vi "Untitled 2.vi"() -> ()   [LabVIEW 2016]
doc: "Приложение для управления четырьмя шаговыми двигателями. Обратной связи с двигателями не имеется."
uses:
  Control 2.ctl
  Control 1.ctl
  Control 3.ctl
  Control 4.ctl
  Control 5.ctl
  <vilib>/Instr/_visa.llb/VISA Configure Serial Port (Instr).vi
panel:
  in  "Stop двигатель 4":T1
  in  "Блокировать счётчик №4":T2
  out "text4":string
  in  "Задать текущее положение нулевым 4":T3
  out "положение шд 4":T4 scale=-10.0..190.0
  in  "Установка шага вращения":i32=1 min=0 max=11400
  in  "Вернуться в нулевое положение 4":bool
  in  "Вращение по минутам - 4":bool
  in  "Вращение по минутам + 4":bool
  out "минуты":string
  out "градусы, минуты":string
  out "положение в мин 4":i32
  in  "stop":T5
  in  "Stop двигатель 3":T1
  in  "Блокировать трубку №3":T2
  out "text3":string
  in  "Задать текущее положение нулевым 3":T3
  out "положение шд 3":T4 scale=-10.0..190.0
  in  "Установка шага вращения":i32=1 min=0 max=11400
  in  "Вернуться в нулевое положение 3":bool
  in  "Вращение по минутам - 3":bool
  in  "Вращение по минутам + 3":bool
  out "минуты":string
  out "градусы, минуты":string
  out "положение в мин 3":i32
  in  "Блокировать стол №2":T2
  out "text2":string
  in  "Stop двигатель 2":T1
  out "положение в мин 2":i32
  out "градусы, минуты":string
  out "минуты":string
  in  "Вращение по минутам + 2":bool
  in  "Вращение по минутам - 2":bool
  in  "Вернуться в нулевое положение 2":bool
  in  "Установка шага вращения":i32=1 min=0 max=11400
  out "положение шд 2":T4 scale=-10.0..190.0
  in  "Задать текущее положение нулевым 2":T3
  in  "Блокировать зеркало №1":bool
  in  "Задать текущее положение нулевым":T3
  out "положение шд":T4 scale=-10.0..190.0
  out "минуты":string
  out "градусы, минуты":string
  in  "Установка шага вращения":i32=1 min=0 max=11400
  out "положение в мин 1":i32
  in  "Stop двигатель":bool
  in  "Вернуться в нулевое положение":bool
  in  "Вращение по минутам -":bool
  in  "Вращение по минутам +":bool
  out "4":i32
  out "3":i32
  out "2":i32
  out "1":i32
  in  "Выберете порт":refnum<visa-resource-name>="COM1"
  # "Поворотный стол №2"
  # "Зеркало №1"
  # "Текущее\nположение"
  # "Текущее\nположение"
  # "Счётчик №4"
  # "Рентгеновская трубка №3"
  # "Текущее\nположение"
  # "Текущее\nположение"
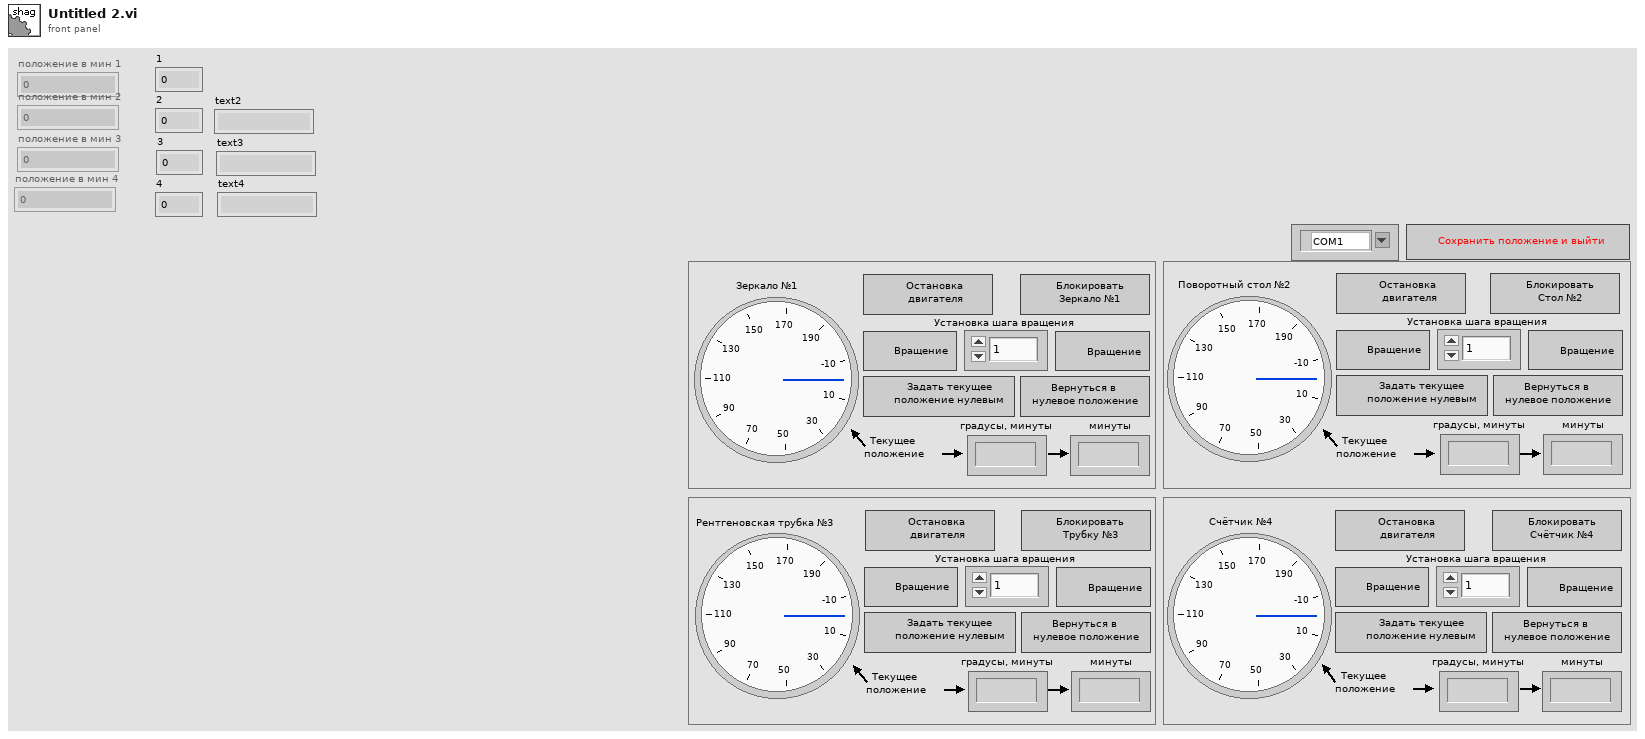
[diagram p1: front panel]
types:
  T1 = typedef "Control 3.ctl" = bool
  T2 = typedef "Control 4.ctl" = bool
  T3 = typedef "Control 1.ctl" = bool
  T4 = typedef "Control 2.ctl" = i32
  T5 = typedef "Control 5.ctl" = bool
  T6 = enum16{"open", "replace", "create", "open or create", "replace or create", "replace or create with confirmation"}
  T7 = enum8{"Enabled", "Disabled", "Disabled and Grayed Out"}
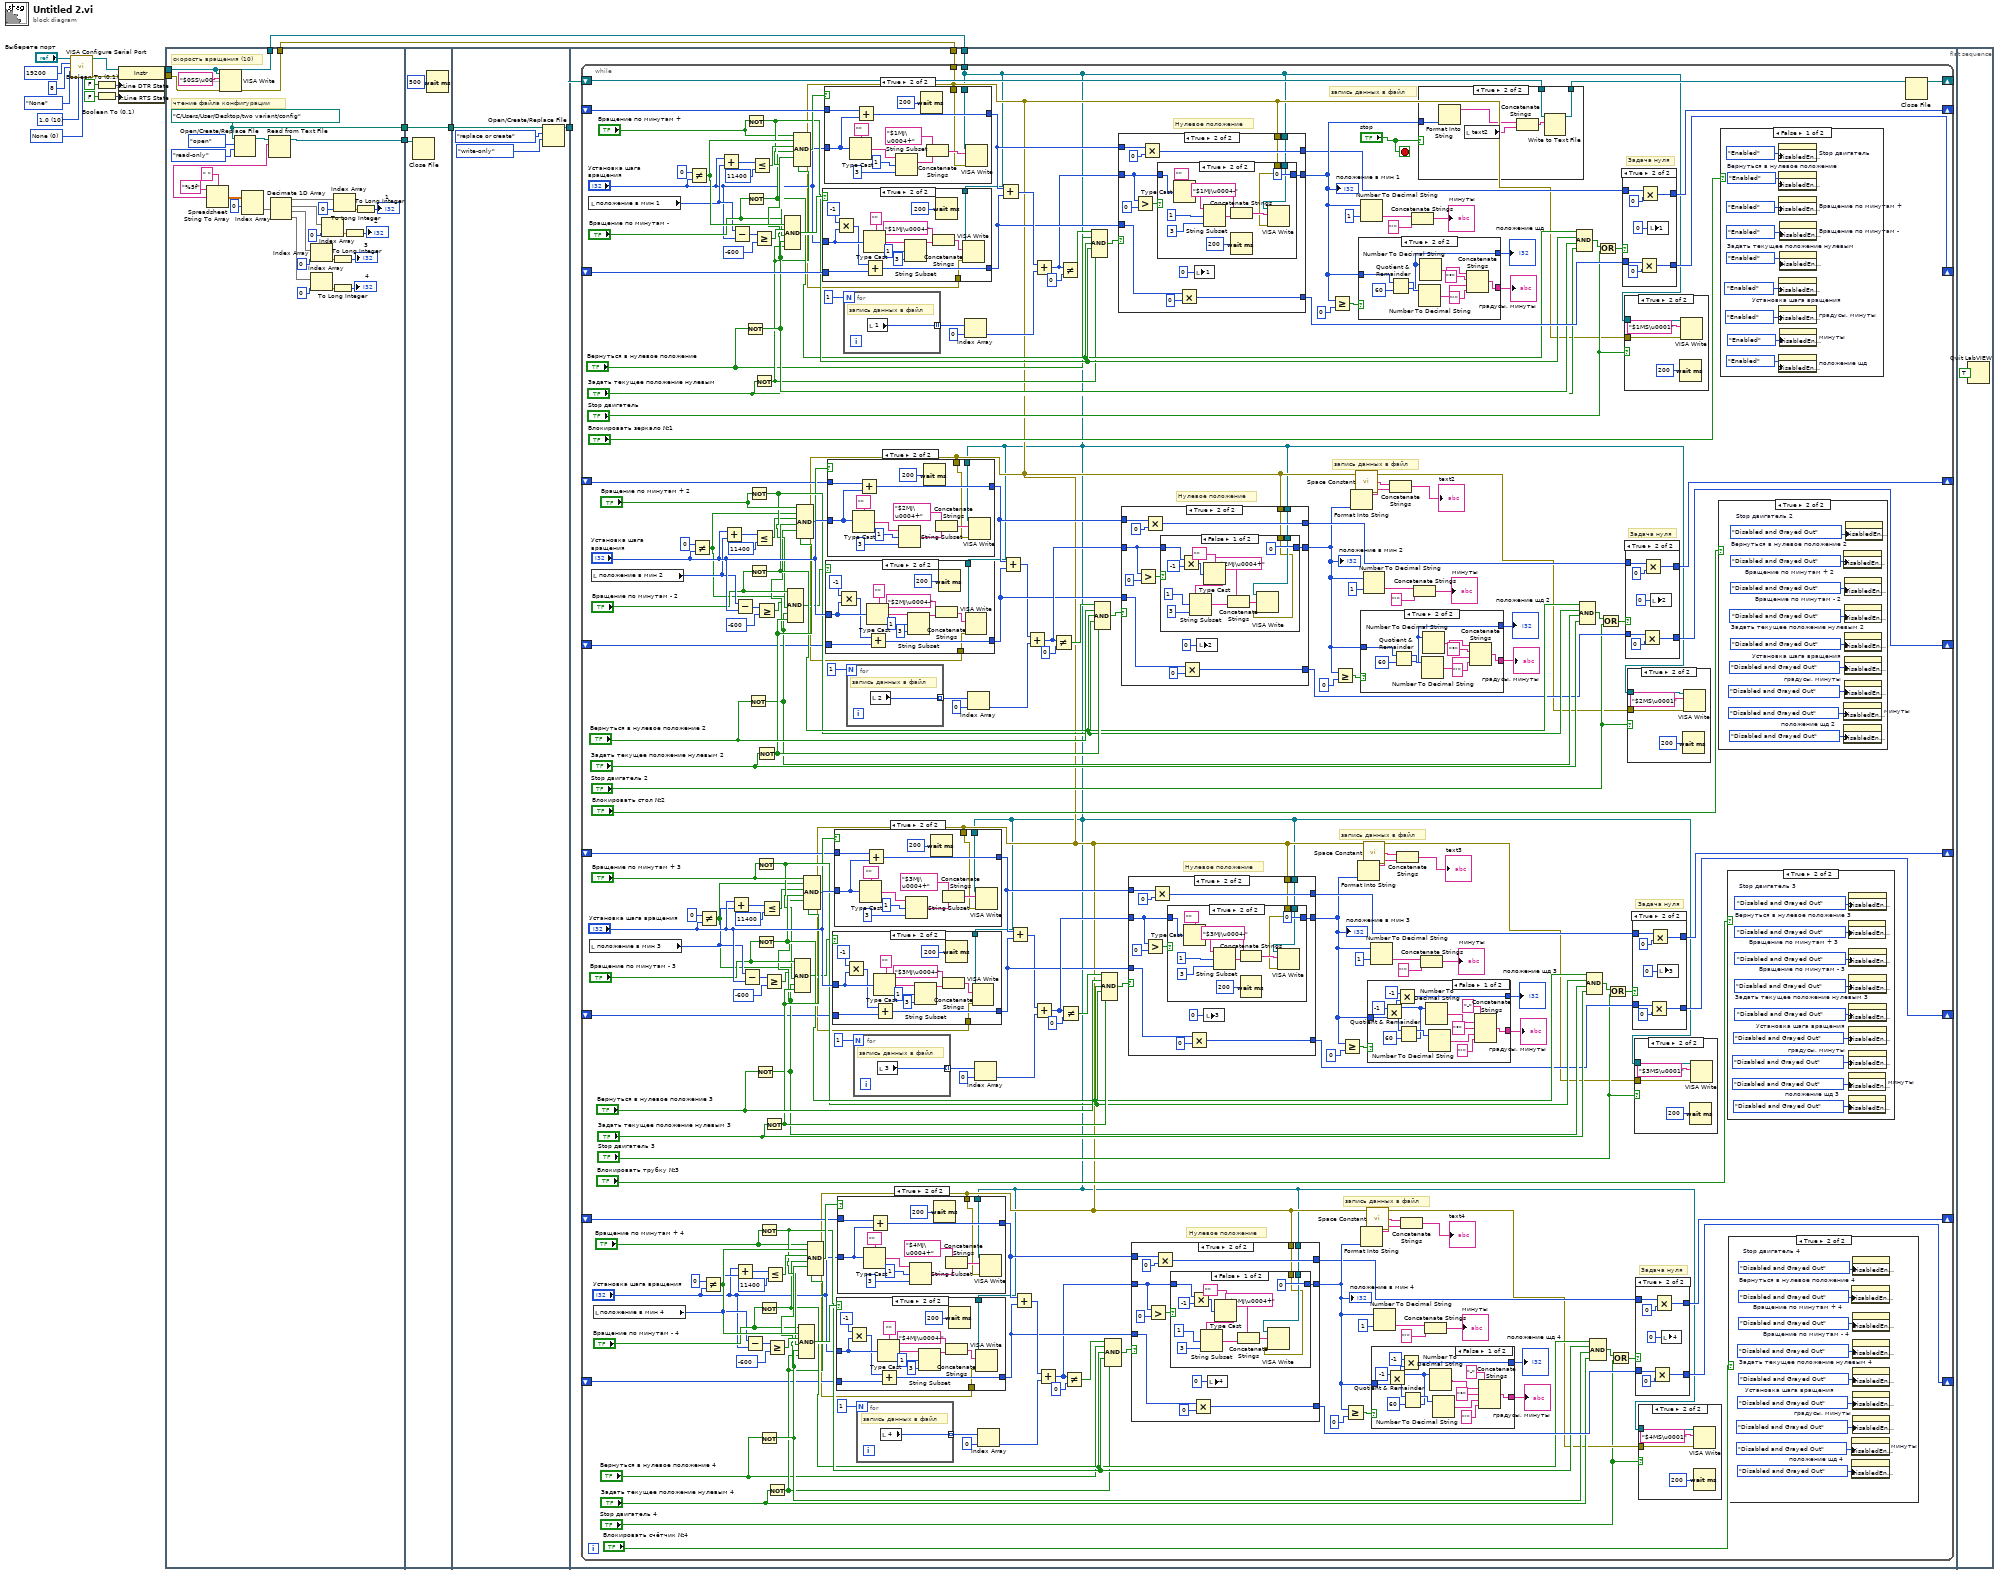
[diagram p0: block diagram]
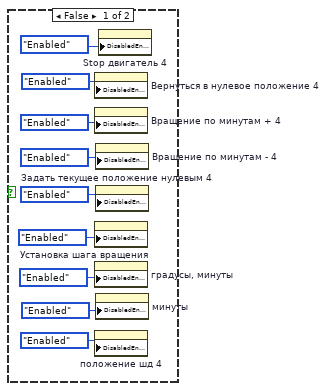
[diagram p2: hidden frame]
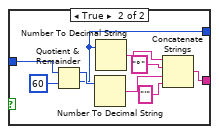
[diagram p5: hidden frame]
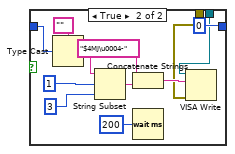
[diagram p7: hidden frame]
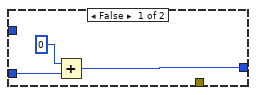
[diagram p8: hidden frame]
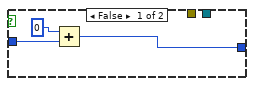
[diagram p9: hidden frame]
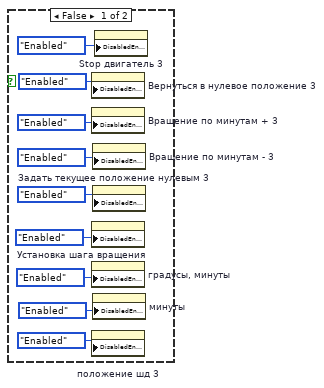
[diagram p10: hidden frame]
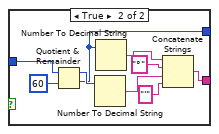
[diagram p13: hidden frame]
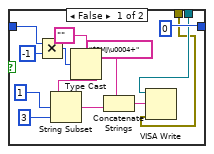
[diagram p15: hidden frame]
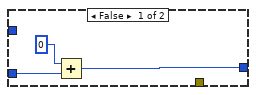
[diagram p16: hidden frame]
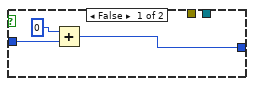
[diagram p17: hidden frame]
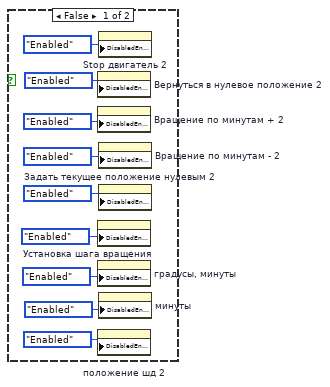
[diagram p18: hidden frame]
diagram:
  w9 = u16 0 items=["None"=0, "XON/XOFF"=1, "RTS/CTS"=2, "DTR/DSR"=4] ("Контроль переполнения")
  w10 = u16 10 items=["1.0"=10, "1.5"=15, "2.0"=20] ("Стоповый бит")
  w13 = u32 19200 items=["9600"=9600, "19200"=19200, "38400"=38400, "57600"=57600] ("Скорость обмена данными")
  n1 = call-poly "VISA Configure Serial Port"("VISA resource name"="Выберете порт", "baud rate (9600)"=w13, "data bits (8)"=u16 8 ("Число бит на символ"), "parity (0:none)"=enum16{"None", "Odd", "Even", "Mark", "Space"}."None" ("Контроль чётности"), "stop bits (10: 1 bit)"=w10, "flow control (0:none)"=w9) -> ("VISA resource name out"=w18:refnum<visa-resource-name>, "error out"=w17:errorcluster)  [unwired: 8 in]
  n2 = Boolean To (0,1)(Boolean=FALSE ("DTR Write")) -> (0, 1=w19:i16)
  n3 = Boolean To (0,1)(Boolean=FALSE ("DTR Write")) -> (0, 1=w20:i16)
  n4 = property class="Instr"(reference=w18, error in=w17, "Serial Settings:Modem Line Settings:Line DTR State"=w19, "Serial Settings:Modem Line Settings:Line RTS State"=w20) -> (reference out=w8:refnum<visa-resource-name>, error out=w7:errorcluster)
  n5 = flat-sequence {
    tunnel: w8 -> [w23]
    tunnel: w7 -> [w22]
    tunnel: [w24] -> w6
    tunnel: [w23] -> w1
    tunnel: [w22] -> w2
    tunnel: [w21] -> w5
    tunnel: w6 -> [w52]
    tunnel: w5 -> [w51]
    tunnel: [w51] -> w4
    tunnel: w4 -> [w55]
    tunnel: [w54] -> w3
    tunnel: w3 -> [w61]
    tunnel: w2 -> [w58]
    tunnel: w1 -> [w59]
    frame #0 {
      w21 = path "C:/Users/User/Desktop/two variant/config"
      # "чтение файла конфигурации"
      # "скорость вращения (10)"
      n6 = VISA Write(VISA resource name=w23, write buffer="$0SS\u0001\u0010", error in (no error)=w22) -> ()  [unwired: 3 out]
      n7 = Open/Create/Replace File(file path (use dialog)=w21, operation (0:open)=T6."open", access (0:read/write)=enum16{"read/write", "read-only", "write-only"}."read-only") -> (refnum out=w47:refnum<file>)  [unwired: 3 in, 2 out]
      n8 = Read from Text File(file (use dialog)=w47) -> (refnum out=w24:refnum<file>, text=w34:string)  [unwired: 3 in, 2 out]
      n9 = Spreadsheet String To Array(delimiter (Tab)=" ", format string="%5f", spreadsheet string=w34) -> (array=w44:dbl[][])  [unwired: 1 in]
      n10 = Index Array(array=w44, index (row)=0 ("index")) -> (element=w42:dbl[])  [unwired: 1 in]
      n11 = Decimate 1D Array(w42) -> (w39:dbl[], w30:dbl[], w29:dbl[], w25:dbl[])
      n12 = Index Array(array=w29, index=0) -> (element=w32:dbl)
      n13 = Index Array(array=w25, index=0) -> (element=w27:dbl)
      n14 = Index Array(array=w30, index=0) -> (element=w38:dbl)
      n15 = To Long Integer(number=w32) -> (32bit integer=→"3":i32)
      n16 = To Long Integer(number=w27) -> (32bit integer=→"4":i32)
      n17 = Index Array(array=w39, index=0) -> (element=w37:dbl)
      n18 = To Long Integer(number=w38) -> (32bit integer=→"2":i32)
      n19 = To Long Integer(number=w37) -> (32bit integer=→"1":i32)
    }
    frame #1 {
      n20 = Close File(refnum=w52) -> ()  [unwired: 1 in, 2 out]
      n21 = Wait (ms)(milliseconds to wait=u32 500) -> ()  [unwired: 1 out]
    }
    frame #2 {
      n22 = Open/Create/Replace File(file path (use dialog)=w55, operation (0:open)=T6."replace or create", access (0:read/write)=enum16{"read/write", "read-only", "write-only"}."write-only") -> (refnum out=w54:refnum<file>)  [unwired: 3 in, 2 out]
    }
    frame #3 {
      n23 = while {
        shift-right: [w245] -> w60
        shift-left: w61 -> [w246]
        shift-right: [w241] -> _
        shift-left: _ -> [w275]
        shift-right: [w240] -> _
        shift-left: _ -> [w269]
        tunnel: w59 -> [w64]
        tunnel: w58 -> [w65]
        shift-right: [w177] -> _
        shift-left: _ -> [w179]
        shift-right: [w176] -> _
        shift-left: _ -> [w178]
        shift-right: [w121] -> _
        shift-left: _ -> [w123]
        shift-right: [w120] -> _
        shift-left: _ -> [w122]
        shift-right: [w67] -> _
        shift-left: _ -> [w69]
        shift-right: [w66] -> _
        shift-left: _ -> [w68]
        stop <- "stop" stop-if-true
        # "Задача нуля"
        # "запись данных в файл"
        # "Нулевое положение"
        # "Задача нуля"
        # "запись данных в файл"
        # "Нулевое положение"
        # "Задача нуля"
        # "запись данных в файл"
        # "Нулевое положение"
        # "Задача нуля"
        # "запись данных в файл"
        # "Нулевое положение"
        n24 = local read "положение в мин 1"() -> (w227:i32)
        n25 = local read "положение в мин 3"() -> (w168:i32)
        n26 = local read "положение в мин 2"() -> (w221:i32)
        n27 = local read "положение в мин 4"() -> (w72:i32)
        n28 = Not Equal?(x=0 ("y"), y="Установка шага вращения") -> (x != y?=w268:bool)
        n29 = Not Equal?(x=0 ("y"), y="Установка шага вращения") -> (x != y?=w185:bool)
        n30 = Not Equal?(x=0 ("y"), y="Установка шага вращения") -> (x != y?=w132:bool)
        n31 = Not Equal?(x=0 ("y"), y="Установка шага вращения") -> (x != y?=w108:bool)
        n32 = Add(x="Установка шага вращения", y=w227) -> (x+y=w273:i32)
        n33 = Add(x="Установка шага вращения", y=w221) -> (x+y=w181:i32)
        n34 = Add(x="Установка шага вращения", y=w168) -> (x+y=w128:i32)
        n35 = Subtract(x=w227, y="Установка шага вращения") -> (x-y=w228:i32)
        n36 = Subtract(x=w221, y="Установка шага вращения") -> (x-y=w220:i32)
        n37 = Add(x="Установка шага вращения", y=w72) -> (x+y=w112:i32)
        n38 = Subtract(x=w168, y="Установка шага вращения") -> (x-y=w167:i32)
        n39 = Not(x="Вернуться в нулевое положение") -> (.not. x?=w239:bool)
        n40 = Subtract(x=w72, y="Установка шага вращения") -> (x-y=w73:i32)
        n41 = Not(x="Вращение по минутам +") -> (.not. x?=w238:bool)
        n42 = Not(x="Вращение по минутам -") -> (.not. x?=w237:bool)
        n43 = Not(x="Вернуться в нулевое положение 2") -> (.not. x?=w210:bool)
        n44 = Not(x="Вращение по минутам + 2") -> (.not. x?=w211:bool)
        n45 = Not(x="Вращение по минутам - 2") -> (.not. x?=w212:bool)
        n46 = Less Or Equal?(x=w273, y=11400) -> (x <= y?=w272:bool)
        n47 = Greater Or Equal?(x=w228, y=-600) -> (x >= y?=w266:bool)
        n48 = Not(x="Задать текущее положение нулевым") -> (.not. x?=w236:T3)
        n49 = Less Or Equal?(x=w181, y=11400) -> (x <= y?=w182:bool)
        n50 = Not(x="Вернуться в нулевое положение 3") -> (.not. x?=w157:bool)
        n51 = Not(x="Вращение по минутам + 3") -> (.not. x?=w158:bool)
        n52 = Not(x="Вращение по минутам - 3") -> (.not. x?=w159:bool)
        n53 = Greater Or Equal?(x=w220, y=-600) -> (x >= y?=w187:bool)
        n54 = Not(x="Задать текущее положение нулевым 2") -> (.not. x?=w213:T3)
        n55 = Not(x="Вернуться в нулевое положение 4") -> (.not. x?=w83:bool)
        n56 = Not(x="Вращение по минутам + 4") -> (.not. x?=w82:bool)
        n57 = Not(x="Вращение по минутам - 4") -> (.not. x?=w81:bool)
        n58 = Less Or Equal?(x=w128, y=11400) -> (x <= y?=w129:bool)
        n59 = Greater Or Equal?(x=w167, y=-600) -> (x >= y?=w134:bool)
        n60 = Not(x="Задать текущее положение нулевым 3") -> (.not. x?=w160:T3)
        n61 = Less Or Equal?(x=w112, y=11400) -> (x <= y?=w111:bool)
        n62 = Greater Or Equal?(x=w73, y=-600) -> (x >= y?=w106:bool)
        n63 = Not(x="Задать текущее положение нулевым 4") -> (.not. x?=w80:T3)
        n64 = Compound Arithmetic op=AND("Вращение по минутам -", w268, w266, w238, w239, w236) -> (w265:T3)
        n65 = Compound Arithmetic op=AND("Вращение по минутам - 2", w185, w187, w211, w210, w213) -> (w188:T3)
        n66 = Compound Arithmetic op=AND("Вращение по минутам +", w268, w272, w237, w239, w236) -> (w270:T3)
        n67 = Compound Arithmetic op=AND("Вращение по минутам - 3", w132, w134, w158, w157, w160) -> (w135:T3)
        n68 = Compound Arithmetic op=AND("Вращение по минутам + 2", w185, w182, w212, w210, w213) -> (w184:T3)
        n69 = Compound Arithmetic op=AND("Вращение по минутам - 4", w108, w106, w82, w83, w80) -> (w105:T3)
        n70 = Compound Arithmetic op=AND("Вращение по минутам + 3", w132, w129, w159, w157, w160) -> (w131:T3)
        n71 = Compound Arithmetic op=AND("Вращение по минутам + 4", w108, w111, w81, w83, w80) -> (w109:T3)
        n72 = case shown="True" w265 {
          tunnel: [w770 w779] -> w255
          tunnel: "Установка шага вращения" -> [_ w774]
          tunnel: w269 -> [w769 w775]
          tunnel: w64 -> [_ w777]
          tunnel: w65 -> [_ w776]
          frame False {
            n73 = Add(x=0, y=w769) -> (x+y=w770:i32)
          }
          frame True {
            n74 = Multiply(x=-1, y=w774) -> (x*y=w773:i32)
            n75 = Type Cast(type="", x=w774) -> (*(type *) &x=w782:string)
            n76 = Add(x=w773, y=w775) -> (x+y=w779:i32)
            n77 = String Subset(string=w782, offset (0)=1, length (rest)=3 ("length (rest)")) -> (substring=w781:string)
            n78 = Concatenate Strings("$1MJ\u0004-" ("write buffer"), w781) -> (w785:string)
            n79 = Wait (ms)(milliseconds to wait=u32 200) -> ()  [unwired: 1 out]
            n80 = VISA Write(VISA resource name=w777, write buffer=w785, error in (no error)=w776) -> ()  [unwired: 3 out]
          }
        }
        n81 = case shown="True" w270 {
          tunnel: [w788 w795] -> w256
          tunnel: "Установка шага вращения" -> [_ w794]
          tunnel: w275 -> [w787 w791]
          tunnel: w64 -> [_ w793]
          tunnel: w65 -> [_ w792]
          frame False {
            n82 = Add(x=0, y=w787) -> (x+y=w788:i32)
          }
          frame True {
            n83 = Type Cast(type="", x=w794) -> (*(type *) &x=w798:string)
            n84 = Add(x=w791, y=w794) -> (x+y=w795:i32)
            n85 = String Subset(string=w798, offset (0)=1, length (rest)=3 ("length (rest)")) -> (substring=w797:string)
            n86 = Wait (ms)(milliseconds to wait=u32 200) -> ()  [unwired: 1 out]
            n87 = Concatenate Strings("$1MJ\u0004+" ("write buffer"), w797) -> (w801:string)
            n88 = VISA Write(VISA resource name=w793, write buffer=w801, error in (no error)=w792) -> ()  [unwired: 3 out]
          }
        }
        n89 = case shown="True" w188 {
          tunnel: [w633 w642] -> w198
          tunnel: "Установка шага вращения" -> [_ w637]
          tunnel: w178 -> [w632 w638]
          tunnel: w64 -> [_ w640]
          tunnel: w65 -> [_ w639]
          frame False {
            n90 = Add(x=0, y=w632) -> (x+y=w633:i32)
          }
          frame True {
            n91 = Multiply(x=-1, y=w637) -> (x*y=w636:i32)
            n92 = Type Cast(type="", x=w637) -> (*(type *) &x=w645:string)
            n93 = Add(x=w636, y=w638) -> (x+y=w642:i32)
            n94 = String Subset(string=w645, offset (0)=1, length (rest)=3 ("length (rest)")) -> (substring=w644:string)
            n95 = Concatenate Strings("$2MJ\u0004-" ("write buffer"), w644) -> (w648:string)
            n96 = Wait (ms)(milliseconds to wait=u32 200) -> ()  [unwired: 1 out]
            n97 = VISA Write(VISA resource name=w640, write buffer=w648, error in (no error)=w639) -> ()  [unwired: 3 out]
          }
        }
        n98 = case shown="True" w184 {
          tunnel: [w651 w658] -> w197
          tunnel: "Установка шага вращения" -> [_ w657]
          tunnel: w179 -> [w650 w654]
          tunnel: w64 -> [_ w656]
          tunnel: w65 -> [_ w655]
          frame False {
            n99 = Add(x=0, y=w650) -> (x+y=w651:i32)
          }
          frame True {
            n100 = Type Cast(type="", x=w657) -> (*(type *) &x=w661:string)
            n101 = Add(x=w654, y=w657) -> (x+y=w658:i32)
            n102 = String Subset(string=w661, offset (0)=1, length (rest)=3 ("length (rest)")) -> (substring=w660:string)
            n103 = Wait (ms)(milliseconds to wait=u32 200) -> ()  [unwired: 1 out]
            n104 = Concatenate Strings("$2MJ\u0004+" ("write buffer"), w660) -> (w664:string)
            n105 = VISA Write(VISA resource name=w656, write buffer=w664, error in (no error)=w655) -> ()  [unwired: 3 out]
          }
        }
        n106 = case shown="True" w135 {
          tunnel: [w503 w512] -> w145
          tunnel: "Установка шага вращения" -> [_ w507]
          tunnel: w122 -> [w502 w508]
          tunnel: w64 -> [_ w510]
          tunnel: w65 -> [_ w509]
          frame False {
            n107 = Add(x=0, y=w502) -> (x+y=w503:i32)
          }
          frame True {
            n108 = Multiply(x=-1, y=w507) -> (x*y=w506:i32)
            n109 = Type Cast(type="", x=w507) -> (*(type *) &x=w515:string)
            n110 = Add(x=w506, y=w508) -> (x+y=w512:i32)
            n111 = String Subset(string=w515, offset (0)=1, length (rest)=3 ("length (rest)")) -> (substring=w514:string)
            n112 = Concatenate Strings("$3MJ\u0004-" ("write buffer"), w514) -> (w518:string)
            n113 = Wait (ms)(milliseconds to wait=u32 200) -> ()  [unwired: 1 out]
            n114 = VISA Write(VISA resource name=w510, write buffer=w518, error in (no error)=w509) -> ()  [unwired: 3 out]
          }
        }
        n115 = case shown="True" w131 {
          tunnel: [w521 w528] -> w144
          tunnel: "Установка шага вращения" -> [_ w527]
          tunnel: w123 -> [w520 w524]
          tunnel: w64 -> [_ w526]
          tunnel: w65 -> [_ w525]
          frame False {
            n116 = Add(x=0, y=w520) -> (x+y=w521:i32)
          }
          frame True {
            n117 = Type Cast(type="", x=w527) -> (*(type *) &x=w531:string)
            n118 = Add(x=w524, y=w527) -> (x+y=w528:i32)
            n119 = String Subset(string=w531, offset (0)=1, length (rest)=3 ("length (rest)")) -> (substring=w530:string)
            n120 = Wait (ms)(milliseconds to wait=u32 200) -> ()  [unwired: 1 out]
            n121 = Concatenate Strings("$3MJ\u0004+" ("write buffer"), w530) -> (w534:string)
            n122 = VISA Write(VISA resource name=w526, write buffer=w534, error in (no error)=w525) -> ()  [unwired: 3 out]
          }
        }
        n123 = case shown="True" w105 {
          tunnel: [w373 w382] -> w95
          tunnel: "Установка шага вращения" -> [_ w377]
          tunnel: w68 -> [w372 w378]
          tunnel: w64 -> [_ w380]
          tunnel: w65 -> [_ w379]
          frame False {
            n124 = Add(x=0, y=w372) -> (x+y=w373:i32)
          }
          frame True {
            n125 = Multiply(x=-1, y=w377) -> (x*y=w376:i32)
            n126 = Type Cast(type="", x=w377) -> (*(type *) &x=w385:string)
            n127 = Add(x=w376, y=w378) -> (x+y=w382:i32)
            n128 = String Subset(string=w385, offset (0)=1, length (rest)=3 ("length (rest)")) -> (substring=w384:string)
            n129 = Concatenate Strings("$4MJ\u0004-" ("write buffer"), w384) -> (w388:string)
            n130 = Wait (ms)(milliseconds to wait=u32 200) -> ()  [unwired: 1 out]
            n131 = VISA Write(VISA resource name=w380, write buffer=w388, error in (no error)=w379) -> ()  [unwired: 3 out]
          }
        }
        n132 = case shown="True" w109 {
          tunnel: [w391 w398] -> w96
          tunnel: "Установка шага вращения" -> [_ w397]
          tunnel: w69 -> [w390 w394]
          tunnel: w64 -> [_ w396]
          tunnel: w65 -> [_ w395]
          frame False {
            n133 = Add(x=0, y=w390) -> (x+y=w391:i32)
          }
          frame True {
            n134 = Type Cast(type="", x=w397) -> (*(type *) &x=w401:string)
            n135 = Add(x=w394, y=w397) -> (x+y=w398:i32)
            n136 = String Subset(string=w401, offset (0)=1, length (rest)=3 ("length (rest)")) -> (substring=w400:string)
            n137 = Wait (ms)(milliseconds to wait=u32 200) -> ()  [unwired: 1 out]
            n138 = Concatenate Strings("$4MJ\u0004+" ("write buffer"), w400) -> (w404:string)
            n139 = VISA Write(VISA resource name=w396, write buffer=w404, error in (no error)=w395) -> ()  [unwired: 3 out]
          }
        }
        n140 = for {
          N: 1 -> [_]
          tunnel: [w768] -> w263 mode=indexing
          # "запись данных в файл"
          n141 = local read "1"() -> (w768:i32)
        }
        n142 = for {
          N: 1 -> [_]
          tunnel: [w631] -> w190 mode=indexing
          # "запись данных в файл"
          n143 = local read "2"() -> (w631:i32)
        }
        n144 = for {
          N: 1 -> [_]
          tunnel: [w501] -> w137 mode=indexing
          # "запись данных в файл"
          n145 = local read "3"() -> (w501:i32)
        }
        n146 = for {
          N: 1 -> [_]
          tunnel: [w371] -> w103 mode=indexing
          # "запись данных в файл"
          n147 = local read "4"() -> (w371:i32)
        }
        n148 = Index Array(array=w263, index=0) -> (element=w261:i32)
        n149 = Index Array(array=w190, index=0) -> (element=w192:i32)
        n150 = Index Array(array=w137, index=0) -> (element=w139:i32)
        n151 = Index Array(array=w103, index=0) -> (element=w101:i32)
        n152 = Add(x=w256, y=w255) -> (x+y=w260:i32)
        n153 = Add(x=w197, y=w198) -> (x+y=w193:i32)
        n154 = Add(x=w144, y=w145) -> (x+y=w140:i32)
        n155 = Add(x=w96, y=w95) -> (x+y=w100:i32)
        n156 = Add(x=w193, y=w192) -> (x+y=w199:i32)
        n157 = Add(x=w260, y=w261) -> (x+y=w254:i32)
        n158 = Add(x=w140, y=w139) -> (x+y=w146:i32)
        n159 = Add(x=w100, y=w101) -> (x+y=w94:i32)
        n160 = Not Equal?(x=w199, y=0) -> (x != y?=w195:bool)
        n161 = Not Equal?(x=w254, y=0) -> (x != y?=w258:bool)
        n162 = Not Equal?(x=w146, y=0) -> (x != y?=w142:bool)
        n163 = Not Equal?(x=w94, y=0) -> (x != y?=w98:bool)
        n164 = Compound Arithmetic op=AND(w258, "Вернуться в нулевое положение", w237, w238, w236) -> (w257:T3)
        n165 = Compound Arithmetic op=AND(w195, "Вернуться в нулевое положение 2", w212, w211, w213) -> (w196:T3)
        n166 = Compound Arithmetic op=AND(w142, "Вернуться в нулевое положение 3", w159, w158, w160) -> (w143:T3)
        n167 = Compound Arithmetic op=AND(w98, "Вернуться в нулевое положение 4", w81, w82, w80) -> (w97:T3)
        n168 = case shown="True" w257 {
          tunnel: [w727 w742] -> w244
          tunnel: [w729 w740] -> w243
          tunnel: [w728 w736] -> w242
          tunnel: w256 -> [w729 w734]
          tunnel: w255 -> [w728 w733]
          tunnel: w254 -> [w727 w732]
          tunnel: w64 -> [_ w731]
          tunnel: w65 -> [_ w730]
          frame False {
          }
          frame True {
            n169 = Greater?(x=w732, y=0) -> (0:w737:bool)
            n170 = Multiply(x=w734, y=0) -> (x*y=w740:i32)
            n171 = case shown="True" w737 {
              tunnel: [0 0] -> w742
              tunnel: w732 -> [w745 w759]
              tunnel: w731 -> [w744 w757]
              tunnel: w730 -> [w743 w758]
              frame False {
                n172 = Multiply(x=w745, y=-1) -> (x*y=w746:i32)
                n173 = Type Cast(type="", x=w746) -> (*(type *) &x=w751:string)
                n174 = String Subset(string=w751, offset (0)=1, length (rest)=3 ("length (rest)")) -> (substring=w750:string)
                n175 = Concatenate Strings("$1MJ\u0004+" ("write buffer"), w750) -> (w754:string)
                n176 = VISA Write(VISA resource name=w744, write buffer=w754, error in (no error)=w743) -> ()  [unwired: 3 out]
              }
              frame True {
                n177 = Type Cast(type="", x=w759) -> (*(type *) &x=w764:string)
                n178 = String Subset(string=w764, offset (0)=1, length (rest)=3 ("length (rest)")) -> (substring=w763:string)
                n179 = Concatenate Strings("$1MJ\u0004-" ("write buffer"), w763) -> (w760:string)
                n180 = Wait (ms)(milliseconds to wait=u32 200) -> ()  [unwired: 1 out]
                n181 = VISA Write(VISA resource name=w757, write buffer=w760, error in (no error)=w758) -> ()  [unwired: 3 out]
              }
            }
            n182 = Multiply(x=w733, y=0) -> (x*y=w736:i32)
            n183 = local write "1"(0 ("1")) -> ()
          }
        }
        "положение в мин 1" <- w244
        n184 = case shown="True" w196 {
          tunnel: [w590 w605] -> w207
          tunnel: [w592 w603] -> w208
          tunnel: [w591 w599] -> w209
          tunnel: w197 -> [w592 w597]
          tunnel: w198 -> [w591 w596]
          tunnel: w199 -> [w590 w595]
          tunnel: w64 -> [_ w594]
          tunnel: w65 -> [_ w593]
          frame False {
          }
          frame True {
            n185 = Greater?(x=w595, y=0) -> (0:w600:bool)
            n186 = Multiply(x=w597, y=0) -> (x*y=w603:i32)
            n187 = case shown="False" w600 {
              tunnel: [0 0] -> w605
              tunnel: w595 -> [w608 w622]
              tunnel: w594 -> [w607 w620]
              tunnel: w593 -> [w606 w621]
              frame False {
                n188 = Multiply(x=w608, y=-1) -> (x*y=w609:i32)
                n189 = Type Cast(type="", x=w609) -> (*(type *) &x=w614:string)
                n190 = String Subset(string=w614, offset (0)=1, length (rest)=3 ("length (rest)")) -> (substring=w613:string)
                n191 = Concatenate Strings("$2MJ\u0004+" ("write buffer"), w613) -> (w617:string)
                n192 = VISA Write(VISA resource name=w607, write buffer=w617, error in (no error)=w606) -> ()  [unwired: 3 out]
              }
              frame True {
                n193 = Type Cast(type="", x=w622) -> (*(type *) &x=w627:string)
                n194 = String Subset(string=w627, offset (0)=1, length (rest)=3 ("length (rest)")) -> (substring=w626:string)
                n195 = Concatenate Strings("$2MJ\u0004-" ("write buffer"), w626) -> (w623:string)
                n196 = Wait (ms)(milliseconds to wait=u32 200) -> ()  [unwired: 1 out]
                n197 = VISA Write(VISA resource name=w620, write buffer=w623, error in (no error)=w621) -> ()  [unwired: 3 out]
              }
            }
            n198 = Multiply(x=w596, y=0) -> (x*y=w599:i32)
            n199 = local write "2"(0 ("1")) -> ()
          }
        }
        "положение в мин 2" <- w207
        n200 = case shown="True" w143 {
          tunnel: [w460 w475] -> w154
          tunnel: [w462 w473] -> w155
          tunnel: [w461 w469] -> w156
          tunnel: w144 -> [w462 w467]
          tunnel: w145 -> [w461 w466]
          tunnel: w146 -> [w460 w465]
          tunnel: w64 -> [_ w464]
          tunnel: w65 -> [_ w463]
          frame False {
          }
          frame True {
            n201 = Greater?(x=w465, y=0) -> (0:w470:bool)
            n202 = Multiply(x=w467, y=0) -> (x*y=w473:i32)
            n203 = case shown="True" w470 {
              tunnel: [0 0] -> w475
              tunnel: w465 -> [w478 w492]
              tunnel: w464 -> [w477 w490]
              tunnel: w463 -> [w476 w491]
              frame False {
                n204 = Multiply(x=w478, y=-1) -> (x*y=w479:i32)
                n205 = Type Cast(type="", x=w479) -> (*(type *) &x=w484:string)
                n206 = String Subset(string=w484, offset (0)=1, length (rest)=3 ("length (rest)")) -> (substring=w483:string)
                n207 = Concatenate Strings("$3MJ\u0004+" ("write buffer"), w483) -> (w487:string)
                n208 = VISA Write(VISA resource name=w477, write buffer=w487, error in (no error)=w476) -> ()  [unwired: 3 out]
              }
              frame True {
                n209 = Type Cast(type="", x=w492) -> (*(type *) &x=w497:string)
                n210 = String Subset(string=w497, offset (0)=1, length (rest)=3 ("length (rest)")) -> (substring=w496:string)
                n211 = Concatenate Strings("$3MJ\u0004-" ("write buffer"), w496) -> (w493:string)
                n212 = Wait (ms)(milliseconds to wait=u32 200) -> ()  [unwired: 1 out]
                n213 = VISA Write(VISA resource name=w490, write buffer=w493, error in (no error)=w491) -> ()  [unwired: 3 out]
              }
            }
            n214 = Multiply(x=w466, y=0) -> (x*y=w469:i32)
            n215 = local write "3"(0 ("1")) -> ()
          }
        }
        "положение в мин 3" <- w154
        n216 = case shown="True" w97 {
          tunnel: [w330 w345] -> w86
          tunnel: [w332 w343] -> w85
          tunnel: [w331 w339] -> w84
          tunnel: w96 -> [w332 w337]
          tunnel: w95 -> [w331 w336]
          tunnel: w94 -> [w330 w335]
          tunnel: w64 -> [_ w334]
          tunnel: w65 -> [_ w333]
          frame False {
          }
          frame True {
            n217 = Greater?(x=w335, y=0) -> (0:w340:bool)
            n218 = Multiply(x=w337, y=0) -> (x*y=w343:i32)
            n219 = case shown="False" w340 {
              tunnel: [0 0] -> w345
              tunnel: w335 -> [w348 w362]
              tunnel: w334 -> [w347 w360]
              tunnel: w333 -> [w346 w361]
              frame False {
                n220 = Multiply(x=w348, y=-1) -> (x*y=w349:i32)
                n221 = Type Cast(type="", x=w349) -> (*(type *) &x=w354:string)
                n222 = String Subset(string=w354, offset (0)=1, length (rest)=3 ("length (rest)")) -> (substring=w353:string)
                n223 = Concatenate Strings("$4MJ\u0004+" ("write buffer"), w353) -> (w357:string)
                n224 = VISA Write(VISA resource name=w347, write buffer=w357, error in (no error)=w346) -> ()  [unwired: 3 out]
              }
              frame True {
                n225 = Type Cast(type="", x=w362) -> (*(type *) &x=w367:string)
                n226 = String Subset(string=w367, offset (0)=1, length (rest)=3 ("length (rest)")) -> (substring=w366:string)
                n227 = Concatenate Strings("$4MJ\u0004-" ("write buffer"), w366) -> (w363:string)
                n228 = Wait (ms)(milliseconds to wait=u32 200) -> ()  [unwired: 1 out]
                n229 = VISA Write(VISA resource name=w360, write buffer=w363, error in (no error)=w361) -> ()  [unwired: 3 out]
              }
            }
            n230 = Multiply(x=w336, y=0) -> (x*y=w339:i32)
            n231 = local write "4"(0 ("1")) -> ()
          }
        }
        "положение в мин 4" <- w86
        n232 = Greater Or Equal?(x=w244, y=0) -> (x >= y?=w253:bool)
        n233 = Greater Or Equal?(x=w207, y=0) -> (x >= y?=w200:bool)
        n234 = Greater Or Equal?(x=w154, y=0) -> (x >= y?=w147:bool)
        n235 = Greater Or Equal?(x=w86, y=0) -> (x >= y?=w93:bool)
        n236 = Format Into String(w207) -> (resulting string=w172:string)  [unwired: 3 in, 1 out]
        n237 = call <vilib>:"Space Constant.vi"() -> ("String"=w173:string)
        n238 = Format Into String(w154) -> (resulting string=w124:string)  [unwired: 3 in, 1 out]
        n239 = case shown="True" w253 {
          tunnel: [w714 w721] -> w247
          tunnel: [w705 w719] -> w230
          tunnel: w244 -> [w704 w718]
          frame False {
            n240 = Multiply(x=-1, y=w704) -> (x*y=w710:i32)
            n241 = Quotient & Remainder(x=w710, y=60) -> (x-y*floor(x/y)=w713:i32, floor(x/y)=w706:i32)
            n242 = Multiply(x=-1, y=w706) -> (x*y=w705:i32)
            n243 = Number To Decimal String(number=w706) -> (decimal integer string=w711:string)  [unwired: 1 in]
            n244 = Number To Decimal String(number=w713) -> (decimal integer string=w712:string)  [unwired: 1 in]
            n245 = Concatenate Strings("-" ("string"), w711, "°" ("string"), w712, "'" ("string")) -> (w714:string)
          }
          frame True {
            n246 = Quotient & Remainder(x=w718, y=60) -> (x-y*floor(x/y)=w720:i32, floor(x/y)=w719:i32)
            n247 = Number To Decimal String(number=w720) -> (decimal integer string=w722:string)  [unwired: 1 in]
            n248 = Number To Decimal String(number=w719) -> (decimal integer string=w723:string)  [unwired: 1 in]
            n249 = Concatenate Strings(w723, "°" ("string"), w722, "'" ("string")) -> (w721:string)
          }
        }
        "градусы, минуты" <- w247
        "положение шд" <- w230
        n250 = Number To Decimal String(number=w244, width (-)=i16 1) -> (decimal integer string=w250:string)
        n251 = case shown="True" w200 {
          tunnel: [w577 w584] -> w206
          tunnel: [w568 w582] -> w218
          tunnel: w207 -> [w567 w581]
          frame False {
            n252 = Multiply(x=-1, y=w567) -> (x*y=w573:i32)
            n253 = Quotient & Remainder(x=w573, y=60) -> (x-y*floor(x/y)=w576:i32, floor(x/y)=w569:i32)
            n254 = Multiply(x=-1, y=w569) -> (x*y=w568:i32)
            n255 = Number To Decimal String(number=w569) -> (decimal integer string=w574:string)  [unwired: 1 in]
            n256 = Number To Decimal String(number=w576) -> (decimal integer string=w575:string)  [unwired: 1 in]
            n257 = Concatenate Strings("-" ("string"), w574, "°" ("string"), w575, "'" ("string")) -> (w577:string)
          }
          frame True {
            n258 = Quotient & Remainder(x=w581, y=60) -> (x-y*floor(x/y)=w583:i32, floor(x/y)=w582:i32)
            n259 = Number To Decimal String(number=w583) -> (decimal integer string=w585:string)  [unwired: 1 in]
            n260 = Number To Decimal String(number=w582) -> (decimal integer string=w586:string)  [unwired: 1 in]
            n261 = Concatenate Strings(w586, "°" ("string"), w585, "'" ("string")) -> (w584:string)
          }
        }
        "градусы, минуты" <- w206
        "положение шд 2" <- w218
        n262 = Format Into String(w86) -> (resulting string=w116:string)  [unwired: 3 in, 1 out]
        n263 = Number To Decimal String(number=w207, width (-)=i16 1) -> (decimal integer string=w203:string)
        n264 = call <vilib>:"Space Constant.vi"() -> ("String"=w125:string)
        n265 = call <vilib>:"Space Constant.vi"() -> ("String"=w115:string)
        n266 = case shown="False" w147 {
          tunnel: [w447 w454] -> w153
          tunnel: [w438 w452] -> w165
          tunnel: w154 -> [w437 w451]
          frame False {
            n267 = Multiply(x=-1, y=w437) -> (x*y=w443:i32)
            n268 = Quotient & Remainder(x=w443, y=60) -> (x-y*floor(x/y)=w446:i32, floor(x/y)=w439:i32)
            n269 = Multiply(x=-1, y=w439) -> (x*y=w438:i32)
            n270 = Number To Decimal String(number=w439) -> (decimal integer string=w444:string)  [unwired: 1 in]
            n271 = Number To Decimal String(number=w446) -> (decimal integer string=w445:string)  [unwired: 1 in]
            n272 = Concatenate Strings("-" ("string"), w444, "°" ("string"), w445, "'" ("string")) -> (w447:string)
          }
          frame True {
            n273 = Quotient & Remainder(x=w451, y=60) -> (x-y*floor(x/y)=w453:i32, floor(x/y)=w452:i32)
            n274 = Number To Decimal String(number=w453) -> (decimal integer string=w455:string)  [unwired: 1 in]
            n275 = Number To Decimal String(number=w452) -> (decimal integer string=w456:string)  [unwired: 1 in]
            n276 = Concatenate Strings(w456, "°" ("string"), w455, "'" ("string")) -> (w454:string)
          }
        }
        "градусы, минуты" <- w153
        "положение шд 3" <- w165
        n277 = Number To Decimal String(number=w154, width (-)=i16 1) -> (decimal integer string=w150:string)
        n278 = case shown="False" w93 {
          tunnel: [w317 w324] -> w87
          tunnel: [w308 w322] -> w75
          tunnel: w86 -> [w307 w321]
          frame False {
            n279 = Multiply(x=-1, y=w307) -> (x*y=w313:i32)
            n280 = Quotient & Remainder(x=w313, y=60) -> (x-y*floor(x/y)=w316:i32, floor(x/y)=w309:i32)
            n281 = Multiply(x=-1, y=w309) -> (x*y=w308:i32)
            n282 = Number To Decimal String(number=w309) -> (decimal integer string=w314:string)  [unwired: 1 in]
            n283 = Number To Decimal String(number=w316) -> (decimal integer string=w315:string)  [unwired: 1 in]
            n284 = Concatenate Strings("-" ("string"), w314, "°" ("string"), w315, "'" ("string")) -> (w317:string)
          }
          frame True {
            n285 = Quotient & Remainder(x=w321, y=60) -> (x-y*floor(x/y)=w323:i32, floor(x/y)=w322:i32)
            n286 = Number To Decimal String(number=w323) -> (decimal integer string=w325:string)  [unwired: 1 in]
            n287 = Number To Decimal String(number=w322) -> (decimal integer string=w326:string)  [unwired: 1 in]
            n288 = Concatenate Strings(w326, "°" ("string"), w325, "'" ("string")) -> (w324:string)
          }
        }
        "градусы, минуты" <- w87
        "положение шд 4" <- w75
        n289 = Number To Decimal String(number=w86, width (-)=i16 1) -> (decimal integer string=w90:string)
        n290 = Concatenate Strings(w173, w172) -> (→"text2":string)
        n291 = Concatenate Strings(w125, w124) -> (→"text3":string)
        n292 = Concatenate Strings(w115, w116) -> (→"text4":string)
        n293 = Concatenate Strings(w250, "'" ("string")) -> (→"минуты":string)
        n294 = Concatenate Strings(w203, "'" ("string")) -> (→"минуты":string)
        n295 = case shown="True" "stop" {
          tunnel: [w697 w703] -> w245
          tunnel: w246 -> [w697 w700]
          tunnel: w244 -> [_ w699]
          frame False {
          }
          frame True {
            n296 = Format Into String(w699) -> (resulting string=w701:string)  [unwired: 3 in, 1 out]
            n297 = local read "text2"() -> (w698:string)
            n298 = Concatenate Strings(w701, w698) -> (w702:string)
            n299 = Write to Text File(file (use dialog)=w700, text=w702) -> (refnum out=w703:refnum<file>)  [unwired: 2 in, 2 out]
          }
        }
        n300 = Concatenate Strings(w150, "'" ("string")) -> (→"минуты":string)
        n301 = Concatenate Strings(w90, "'" ("string")) -> (→"минуты":string)
        n302 = Compound Arithmetic op=AND(w237, w238, w239, "Задать текущее положение нулевым") -> (w234:T3)
        n303 = Compound Arithmetic op=AND(w212, w211, w210, "Задать текущее положение нулевым 2") -> (w215:T3)
        n304 = Compound Arithmetic op=AND(w159, w158, w157, "Задать текущее положение нулевым 3") -> (w162:T3)
        n305 = Compound Arithmetic op=AND(w81, w82, w83, "Задать текущее положение нулевым 4") -> (w78:T3)
        n306 = Or(x=w234, y="Stop двигатель") -> (x .or. y?=w235:T3)
        n307 = Or(x=w215, y="Stop двигатель 2") -> (x .or. y?=w214:T3)
        n308 = Or(x=w162, y="Stop двигатель 3") -> (x .or. y?=w161:T3)
        n309 = Or(x=w78, y="Stop двигатель 4") -> (x .or. y?=w79:T3)
        n310 = case shown="True" w235 {
          tunnel: [w689 w695] -> w241
          tunnel: w243 -> [w689 w696]
          tunnel: w242 -> [w688 w692]
          tunnel: [w688 w691] -> w240
          frame False {
          }
          frame True {
            n311 = Multiply(x=w692, y=0) -> (x*y=w691:i32)
            n312 = Multiply(x=w696, y=0) -> (x*y=w695:i32)
            n313 = local write "1"(0 ("1")) -> ()
          }
        }
        n314 = case shown="True" "Stop двигатель" {
          tunnel: w64 -> [_ w686]
          tunnel: w65 -> [_ w685]
          frame False {
          }
          frame True {
            n315 = Wait (ms)(milliseconds to wait=u32 200) -> ()  [unwired: 1 out]
            n316 = VISA Write(VISA resource name=w686, write buffer="$1MS\u0001", error in (no error)=w685) -> ()  [unwired: 3 out]
          }
        }
        n317 = case shown="True" w214 {
          tunnel: [w559 w565] -> w177
          tunnel: w208 -> [w559 w566]
          tunnel: w209 -> [w558 w562]
          tunnel: [w558 w561] -> w176
          frame False {
          }
          frame True {
            n318 = Multiply(x=w562, y=0) -> (x*y=w561:i32)
            n319 = Multiply(x=w566, y=0) -> (x*y=w565:i32)
            n320 = local write "2"(0 ("1")) -> ()
          }
        }
        n321 = case shown="True" "Stop двигатель 2" {
          tunnel: w64 -> [_ w556]
          tunnel: w65 -> [_ w555]
          frame False {
          }
          frame True {
            n322 = Wait (ms)(milliseconds to wait=u32 200) -> ()  [unwired: 1 out]
            n323 = VISA Write(VISA resource name=w556, write buffer="$2MS\u0001", error in (no error)=w555) -> ()  [unwired: 3 out]
          }
        }
        n324 = case shown="True" w161 {
          tunnel: [w429 w435] -> w121
          tunnel: w155 -> [w429 w436]
          tunnel: w156 -> [w428 w432]
          tunnel: [w428 w431] -> w120
          frame False {
          }
          frame True {
            n325 = Multiply(x=w432, y=0) -> (x*y=w431:i32)
            n326 = Multiply(x=w436, y=0) -> (x*y=w435:i32)
            n327 = local write "3"(0 ("1")) -> ()
          }
        }
        n328 = case shown="True" "Stop двигатель 3" {
          tunnel: w64 -> [_ w426]
          tunnel: w65 -> [_ w425]
          frame False {
          }
          frame True {
            n329 = Wait (ms)(milliseconds to wait=u32 200) -> ()  [unwired: 1 out]
            n330 = VISA Write(VISA resource name=w426, write buffer="$3MS\u0001", error in (no error)=w425) -> ()  [unwired: 3 out]
          }
        }
        n331 = case shown="True" w79 {
          tunnel: [w299 w305] -> w67
          tunnel: w85 -> [w299 w306]
          tunnel: w84 -> [w298 w302]
          tunnel: [w298 w301] -> w66
          frame False {
          }
          frame True {
            n332 = Multiply(x=w302, y=0) -> (x*y=w301:i32)
            n333 = Multiply(x=w306, y=0) -> (x*y=w305:i32)
            n334 = local write "4"(0 ("1")) -> ()
          }
        }
        n335 = case shown="True" "Stop двигатель 4" {
          tunnel: w64 -> [_ w296]
          tunnel: w65 -> [_ w295]
          frame False {
          }
          frame True {
            n336 = Wait (ms)(milliseconds to wait=u32 200) -> ()  [unwired: 1 out]
            n337 = VISA Write(VISA resource name=w296, write buffer="$4MS\u0001", error in (no error)=w295) -> ()  [unwired: 3 out]
          }
        }
        n338 = case shown="True" "Блокировать стол №2" {
          frame False {
            n339 = property on="Вернуться в нулевое положение 2" class="Bool"("DisabledEnum"=T7."Enabled" ("Disabled")) -> ()  [unwired: 2 in, 2 out]
            n340 = property on="Вращение по минутам + 2" class="Bool"("DisabledEnum"=T7."Enabled" ("Disabled")) -> ()  [unwired: 2 in, 2 out]
            n341 = property on="Установка шага вращения" class="DigNum (strict)"("DisabledEnum"=T7."Enabled" ("Disabled")) -> ()  [unwired: 2 in, 2 out]
            n342 = property on="градусы, минуты" class="Str"("DisabledEnum"=T7."Enabled" ("Disabled")) -> ()  [unwired: 2 in, 2 out]
            n343 = property on="положение шд 2" class="Knob (strict)"("DisabledEnum"=T7."Enabled" ("Disabled")) -> ()  [unwired: 2 in, 2 out]
            n344 = property on="Stop двигатель 2" class="Bool"("DisabledEnum"=T7."Enabled" ("Disabled")) -> ()  [unwired: 2 in, 2 out]
            n345 = property on="Вращение по минутам - 2" class="Bool (strict)"("DisabledEnum"=T7."Enabled" ("Disabled")) -> ()  [unwired: 2 in, 2 out]
            n346 = property on="Задать текущее положение нулевым 2" class="Bool"("DisabledEnum"=T7."Enabled" ("Disabled")) -> ()  [unwired: 2 in, 2 out]
            n347 = property on="минуты" class="Str"("DisabledEnum"=T7."Enabled" ("Disabled")) -> ()  [unwired: 2 in, 2 out]
          }
          frame True {
            n348 = property on="Вернуться в нулевое положение 2" class="Bool"("DisabledEnum"=T7."Disabled and Grayed Out" ("Disabled")) -> ()  [unwired: 2 in, 2 out]
            n349 = property on="минуты" class="Str"("DisabledEnum"=T7."Disabled and Grayed Out" ("Disabled")) -> ()  [unwired: 2 in, 2 out]
            n350 = property on="положение шд 2" class="Knob (strict)"("DisabledEnum"=T7."Disabled and Grayed Out" ("Disabled")) -> ()  [unwired: 2 in, 2 out]
            n351 = property on="Вращение по минутам + 2" class="Bool"("DisabledEnum"=T7."Disabled and Grayed Out" ("Disabled")) -> ()  [unwired: 2 in, 2 out]
            n352 = property on="Вращение по минутам - 2" class="Bool (strict)"("DisabledEnum"=T7."Disabled and Grayed Out" ("Disabled")) -> ()  [unwired: 2 in, 2 out]
            n353 = property on="Задать текущее положение нулевым 2" class="Bool"("DisabledEnum"=T7."Disabled and Grayed Out" ("Disabled")) -> ()  [unwired: 2 in, 2 out]
            n354 = property on="Установка шага вращения" class="DigNum (strict)"("DisabledEnum"=T7."Disabled and Grayed Out" ("Disabled")) -> ()  [unwired: 2 in, 2 out]
            n355 = property on="градусы, минуты" class="Str"("DisabledEnum"=T7."Disabled and Grayed Out" ("Disabled")) -> ()  [unwired: 2 in, 2 out]
            n356 = property on="Stop двигатель 2" class="Bool"("DisabledEnum"=T7."Disabled and Grayed Out" ("Disabled")) -> ()  [unwired: 2 in, 2 out]
          }
        }
        n357 = case shown="False" "Блокировать зеркало №1" {
          frame False {
            n358 = property on="Stop двигатель" class="Bool"("DisabledEnum"=T7."Enabled" ("Disabled")) -> ()  [unwired: 2 in, 2 out]
            n359 = property on="Вернуться в нулевое положение" class="Bool"("DisabledEnum"=T7."Enabled" ("Disabled")) -> ()  [unwired: 2 in, 2 out]
            n360 = property on="Вращение по минутам +" class="Bool"("DisabledEnum"=T7."Enabled" ("Disabled")) -> ()  [unwired: 2 in, 2 out]
            n361 = property on="Установка шага вращения" class="DigNum (strict)"("DisabledEnum"=T7."Enabled" ("Disabled")) -> ()  [unwired: 2 in, 2 out]
            n362 = property on="градусы, минуты" class="Str"("DisabledEnum"=T7."Enabled" ("Disabled")) -> ()  [unwired: 2 in, 2 out]
            n363 = property on="положение шд" class="Knob (strict)"("DisabledEnum"=T7."Enabled" ("Disabled")) -> ()  [unwired: 2 in, 2 out]
            n364 = property on="Вращение по минутам -" class="Bool (strict)"("DisabledEnum"=T7."Enabled" ("Disabled")) -> ()  [unwired: 2 in, 2 out]
            n365 = property on="Задать текущее положение нулевым" class="Bool"("DisabledEnum"=T7."Enabled" ("Disabled")) -> ()  [unwired: 2 in, 2 out]
            n366 = property on="минуты" class="Str"("DisabledEnum"=T7."Enabled" ("Disabled")) -> ()  [unwired: 2 in, 2 out]
          }
          frame True {
            n367 = property on="Вернуться в нулевое положение" class="Bool"("DisabledEnum"=T7."Disabled and Grayed Out" ("Disabled")) -> ()  [unwired: 2 in, 2 out]
            n368 = property on="минуты" class="Str"("DisabledEnum"=T7."Disabled and Grayed Out" ("Disabled")) -> ()  [unwired: 2 in, 2 out]
            n369 = property on="положение шд" class="Knob (strict)"("DisabledEnum"=T7."Disabled and Grayed Out" ("Disabled")) -> ()  [unwired: 2 in, 2 out]
            n370 = property on="Stop двигатель" class="Bool"("DisabledEnum"=T7."Disabled and Grayed Out" ("Disabled")) -> ()  [unwired: 2 in, 2 out]
            n371 = property on="Вращение по минутам +" class="Bool"("DisabledEnum"=T7."Disabled and Grayed Out" ("Disabled")) -> ()  [unwired: 2 in, 2 out]
            n372 = property on="Вращение по минутам -" class="Bool (strict)"("DisabledEnum"=T7."Disabled and Grayed Out" ("Disabled")) -> ()  [unwired: 2 in, 2 out]
            n373 = property on="Задать текущее положение нулевым" class="Bool"("DisabledEnum"=T7."Disabled and Grayed Out" ("Disabled")) -> ()  [unwired: 2 in, 2 out]
            n374 = property on="Установка шага вращения" class="DigNum (strict)"("DisabledEnum"=T7."Disabled and Grayed Out" ("Disabled")) -> ()  [unwired: 2 in, 2 out]
            n375 = property on="градусы, минуты" class="Str"("DisabledEnum"=T7."Disabled and Grayed Out" ("Disabled")) -> ()  [unwired: 2 in, 2 out]
          }
        }
        n376 = case shown="True" "Блокировать трубку №3" {
          frame False {
            n377 = property on="Вернуться в нулевое положение 3" class="Bool"("DisabledEnum"=T7."Enabled" ("Disabled")) -> ()  [unwired: 2 in, 2 out]
            n378 = property on="Вращение по минутам + 3" class="Bool"("DisabledEnum"=T7."Enabled" ("Disabled")) -> ()  [unwired: 2 in, 2 out]
            n379 = property on="Установка шага вращения" class="DigNum (strict)"("DisabledEnum"=T7."Enabled" ("Disabled")) -> ()  [unwired: 2 in, 2 out]
            n380 = property on="градусы, минуты" class="Str"("DisabledEnum"=T7."Enabled" ("Disabled")) -> ()  [unwired: 2 in, 2 out]
            n381 = property on="положение шд 3" class="Knob (strict)"("DisabledEnum"=T7."Enabled" ("Disabled")) -> ()  [unwired: 2 in, 2 out]
            n382 = property on="Вращение по минутам - 3" class="Bool (strict)"("DisabledEnum"=T7."Enabled" ("Disabled")) -> ()  [unwired: 2 in, 2 out]
            n383 = property on="Задать текущее положение нулевым 3" class="Bool"("DisabledEnum"=T7."Enabled" ("Disabled")) -> ()  [unwired: 2 in, 2 out]
            n384 = property on="минуты" class="Str"("DisabledEnum"=T7."Enabled" ("Disabled")) -> ()  [unwired: 2 in, 2 out]
            n385 = property on="Stop двигатель 3" class="Bool"("DisabledEnum"=T7."Enabled" ("Disabled")) -> ()  [unwired: 2 in, 2 out]
          }
          frame True {
            n386 = property on="Вернуться в нулевое положение 3" class="Bool"("DisabledEnum"=T7."Disabled and Grayed Out" ("Disabled")) -> ()  [unwired: 2 in, 2 out]
            n387 = property on="минуты" class="Str"("DisabledEnum"=T7."Disabled and Grayed Out" ("Disabled")) -> ()  [unwired: 2 in, 2 out]
            n388 = property on="положение шд 3" class="Knob (strict)"("DisabledEnum"=T7."Disabled and Grayed Out" ("Disabled")) -> ()  [unwired: 2 in, 2 out]
            n389 = property on="Stop двигатель 3" class="Bool"("DisabledEnum"=T7."Disabled and Grayed Out" ("Disabled")) -> ()  [unwired: 2 in, 2 out]
            n390 = property on="Вращение по минутам + 3" class="Bool"("DisabledEnum"=T7."Disabled and Grayed Out" ("Disabled")) -> ()  [unwired: 2 in, 2 out]
            n391 = property on="Вращение по минутам - 3" class="Bool (strict)"("DisabledEnum"=T7."Disabled and Grayed Out" ("Disabled")) -> ()  [unwired: 2 in, 2 out]
            n392 = property on="Задать текущее положение нулевым 3" class="Bool"("DisabledEnum"=T7."Disabled and Grayed Out" ("Disabled")) -> ()  [unwired: 2 in, 2 out]
            n393 = property on="Установка шага вращения" class="DigNum (strict)"("DisabledEnum"=T7."Disabled and Grayed Out" ("Disabled")) -> ()  [unwired: 2 in, 2 out]
            n394 = property on="градусы, минуты" class="Str"("DisabledEnum"=T7."Disabled and Grayed Out" ("Disabled")) -> ()  [unwired: 2 in, 2 out]
          }
        }
        n395 = case shown="True" "Блокировать счётчик №4" {
          frame False {
            n396 = property on="Вернуться в нулевое положение 4" class="Bool"("DisabledEnum"=T7."Enabled" ("Disabled")) -> ()  [unwired: 2 in, 2 out]
            n397 = property on="Вращение по минутам + 4" class="Bool"("DisabledEnum"=T7."Enabled" ("Disabled")) -> ()  [unwired: 2 in, 2 out]
            n398 = property on="Установка шага вращения" class="DigNum (strict)"("DisabledEnum"=T7."Enabled" ("Disabled")) -> ()  [unwired: 2 in, 2 out]
            n399 = property on="градусы, минуты" class="Str"("DisabledEnum"=T7."Enabled" ("Disabled")) -> ()  [unwired: 2 in, 2 out]
            n400 = property on="положение шд 4" class="Knob (strict)"("DisabledEnum"=T7."Enabled" ("Disabled")) -> ()  [unwired: 2 in, 2 out]
            n401 = property on="Вращение по минутам - 4" class="Bool (strict)"("DisabledEnum"=T7."Enabled" ("Disabled")) -> ()  [unwired: 2 in, 2 out]
            n402 = property on="Задать текущее положение нулевым 4" class="Bool"("DisabledEnum"=T7."Enabled" ("Disabled")) -> ()  [unwired: 2 in, 2 out]
            n403 = property on="минуты" class="Str"("DisabledEnum"=T7."Enabled" ("Disabled")) -> ()  [unwired: 2 in, 2 out]
            n404 = property on="Stop двигатель 4" class="Bool"("DisabledEnum"=T7."Enabled" ("Disabled")) -> ()  [unwired: 2 in, 2 out]
          }
          frame True {
            n405 = property on="Вернуться в нулевое положение 4" class="Bool"("DisabledEnum"=T7."Disabled and Grayed Out" ("Disabled")) -> ()  [unwired: 2 in, 2 out]
            n406 = property on="минуты" class="Str"("DisabledEnum"=T7."Disabled and Grayed Out" ("Disabled")) -> ()  [unwired: 2 in, 2 out]
            n407 = property on="положение шд 4" class="Knob (strict)"("DisabledEnum"=T7."Disabled and Grayed Out" ("Disabled")) -> ()  [unwired: 2 in, 2 out]
            n408 = property on="Stop двигатель 4" class="Bool"("DisabledEnum"=T7."Disabled and Grayed Out" ("Disabled")) -> ()  [unwired: 2 in, 2 out]
            n409 = property on="Вращение по минутам + 4" class="Bool"("DisabledEnum"=T7."Disabled and Grayed Out" ("Disabled")) -> ()  [unwired: 2 in, 2 out]
            n410 = property on="Вращение по минутам - 4" class="Bool (strict)"("DisabledEnum"=T7."Disabled and Grayed Out" ("Disabled")) -> ()  [unwired: 2 in, 2 out]
            n411 = property on="Задать текущее положение нулевым 4" class="Bool"("DisabledEnum"=T7."Disabled and Grayed Out" ("Disabled")) -> ()  [unwired: 2 in, 2 out]
            n412 = property on="Установка шага вращения" class="DigNum (strict)"("DisabledEnum"=T7."Disabled and Grayed Out" ("Disabled")) -> ()  [unwired: 2 in, 2 out]
            n413 = property on="градусы, минуты" class="Str"("DisabledEnum"=T7."Disabled and Grayed Out" ("Disabled")) -> ()  [unwired: 2 in, 2 out]
          }
        }
      }
      n414 = Close File(refnum=w60) -> ()  [unwired: 1 in, 2 out]
    }
    frame #4 {
      n415 = Quit LabVIEW(quit? (T)=TRUE) -> ()
    }
  }
